vi "sub_CRC8.vi"(4 "message":string) -> (1 "CRC8":u8 format="%x")   [LabVIEW 2012]
doc: "This VI computes a CRC16 checksum from <B>message</B>.\nFor compatibility with the MODbus protocol the hi and low bytes of the CRC are swapped."
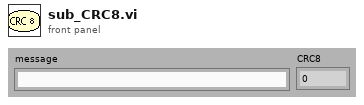
[diagram p1: front panel]
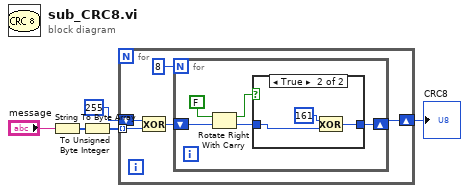
[diagram p0: block diagram]
diagram:
  n1 = String To Byte Array(string="message") -> (unsigned byte array=w4:u8[])
  n2 = To Unsigned Byte Integer(number=w4) -> (unsigned 8bit integer=w2:u8[])
  n3 = for {
    shift-right: [w7] -> w1
    shift-left: u8 255 -> [w8]
    tunnel: w2 -> [w6] mode=indexing
    n4 = Exclusive Or(1:w6, 2:w8) -> (0:w9:u8)
    n5 = for {
      N: 8 -> [_]
      shift-right: [w14] -> w7
      shift-left: w9 -> [w13]
      n6 = Rotate Right With Carry(2:w13, 3:FALSE ("Übertrag")) -> (0:w15:u8, 1:w12:bool)
      n7 = case shown="True" w12 {
        tunnel: w15 -> [w16 w18]
        tunnel: [w16 w17] -> w14
        frame False {
        }
        frame True {
          n8 = Exclusive Or(1:w18, 2:u8 161) -> (0:w17:u8)
        }
      }
    }
  }
  "CRC8" <- w1
